vi "Trigger AI Acquisition.vi"() -> ()   [LabVIEW 2012]
doc: "该范例演示了如果使用DAQmx设备连续采集带缓冲的电压信号。\n\n关于如何连接信号至DAQ设备，请查看设备文档。"
uses:
  <vilib>/DAQmx/read.llb/DAQmx Read (Analog 1D Wfm NChan NSamp).vi
  <vilib>/DAQmx/create/channels.llb/DAQmx Create Channel (AI-Voltage-Basic).vi
  <vilib>/DAQmx/configure/timing.llb/DAQmx Timing (Sample Clock).vi
  <vilib>/DAQmx/configure/task.llb/DAQmx Configure Logging (TDMS).vi
  <vilib>/DAQmx/configure/trigger.llb/DAQmx Start Trigger (Digital Edge).vi
  <vilib>/DAQmx/miscellaneous.llb/DAQmx Fill In Error Info.vi
  <resource>/objmgr/daqmx.rc
panel:
  in  "边沿":i32(ring)=10280 items=["上升"=10280, "下降"=10171]
  in  "源":tag="/Dev1/PFI1"
  in  "停止":bool
  out "波形图":waveform(dbl)[](graph)=[{"t0"=timestamp(3423073651.7132955 s since 1904-01-01), "dt"=0.001, "Y"=array[1000 elements], "attributes"=variant("NI_ChannelName"=variant(string "Dev1/ai1"), "NI_UnitDescription"=variant(string "Volts"))}]
  in  "TDMS文件路径":path
  in  "每个循环采样点":i32=1000
  in  "采样率":dbl=1000.0
  in  "采样时钟源":tag="OnboardClock"
  in  "接线端配置":i32(ring)=-1 items=["默认"=-1, "RSE"=10083, "NRSE"=10078, "差分"=10106, "伪差分"=12529]
  in  "最大电压":dbl=1.0
  in  "最小电压":dbl=-1.0
  in  "物理通道":tag="Dev1/ai1"
  out "实际采样率":dbl=1000.0 format="%0.2f"
  in  "记录模式":i32(ring)=10231 items=["关"=10231, "记录并读取"=15842]
  # "通道设置"
  # "触发设置"
  # "采集数据"
  # "定时设置"
  # "记录设置"
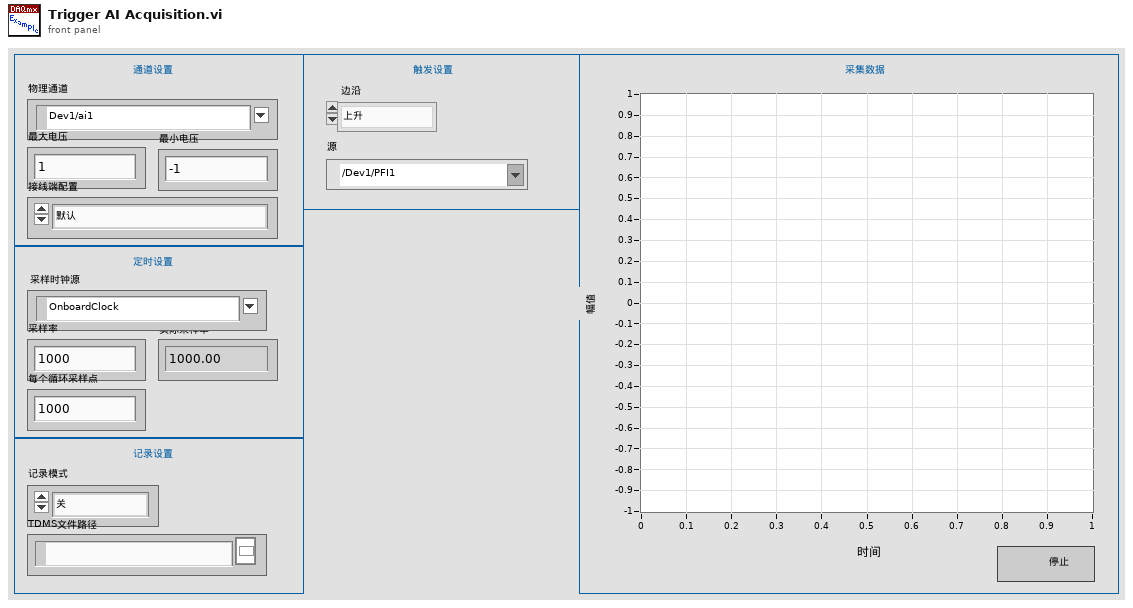
[diagram p1: front panel]
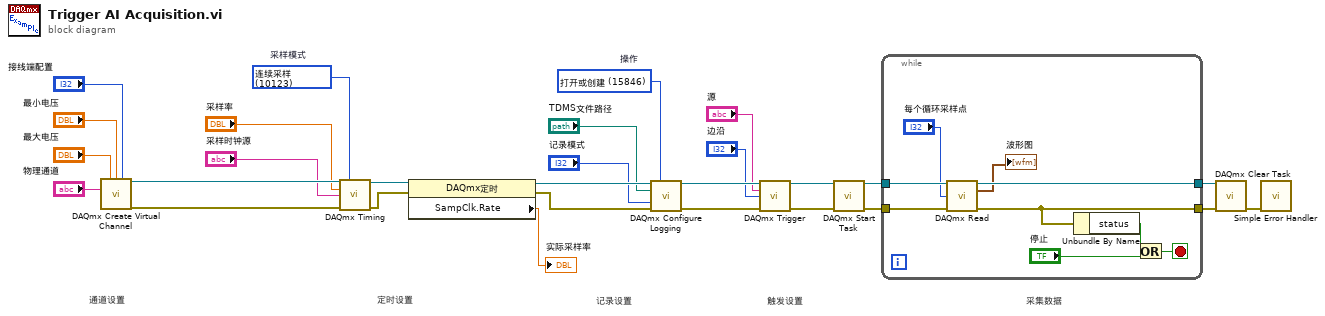
[diagram p0: block diagram]
diagram:
  w1 = 15846 items=["打开"=10437, "打开或创建"=15846, "创建或替换"=15847, "创建"=15848]  # 操作
  w2 = 10123 items=["有限采样"=10178, "连续采样"=10123, "硬件定时单点"=12522]  # 采样模式
  # "触发设置"
  # "采集数据"
  # "定时设置"
  # "通道设置"
  # "记录设置"
  n1 = call-poly <vilib>:"DAQmx Create Virtual Channel.vi"("maximum value"="最大电压", "minimum value"="最小电压", "input terminal configuration"="接线端配置", "physical channels"="物理通道") -> ("task out"=w25:refnum<k21>, "error out"=w26:errorcluster)  [unwired: 10 in]
  n2 = call-poly <vilib>:"DAQmx Timing.vi"("task/channels in"=w25, "sample mode"=w2, "rate"="采样率", "source"="采样时钟源", "error in"=w26) -> ("task out"=w28:refnum<k21>, "error out"=w27:errorcluster)  [unwired: 9 in]
  n3 = property on="属性节点" class="DAQmx定时"(reference=w28, error in=w27) -> (reference out=w24:refnum<k21>, error out=w23:errorcluster, "SampClk.Rate"=→"实际采样率":dbl)
  n4 = call-poly <vilib>:"DAQmx Configure Logging.vi"("task/channels in"=w24, "operation"=w1, "file path"="TDMS文件路径", "logging mode"="记录模式", "error in"=w23) -> ("task out"=w8:refnum<k21>, "error out"=w6:errorcluster)  [unwired: 9 in]
  n5 = call-poly <vilib>:"DAQmx Trigger.vi"("task/channels in"=w8, "source"="源", "edge"="边沿", "error in"=w6) -> ("task out"=w7:refnum<k21>, "error out"=w5:errorcluster)  [unwired: 10 in]
  n6 = call <vilib>:"DAQmx Start Task.vi"("task/channels in"=w7, "error in"=w5) -> ("task out"=w22:refnum<k21>, "error out"=w21:errorcluster)  [unwired: 12 in]
  n7 = while {
    tunnel: w22 -> [w37]
    tunnel: w21 -> [w36]
    tunnel: [w33] -> w19
    tunnel: [w34] -> w20
    stop <- w35 stop-if-true
    n8 = call-poly <vilib>:"DAQmx Read.vi"("task/channels in"=w37, "number of samples per channel"="每个循环采样点", "error in"=w36) -> ("task out"=w34:refnum<k21>, "data"=→"波形图":waveform(dbl)[], "error out"=w33:errorcluster)  [unwired: 10 in]
    n9 = Unbundle By Name ("按名称解除捆绑")(w33) -> ("status"=w32:bool)
    n10 = Or ("或")(x=w32, y="停止") -> (x .or. y?=w35:bool)
  }
  n11 = call <vilib>:"DAQmx Clear Task.vi"("task in"=w20, "error in"=w19) -> ("error out"=w18:errorcluster)  [unwired: 13 in]
  n12 = call <vilib>:"Simple Error Handler.vi"("error in (no error)"=w18) -> ()  [unwired: 4 in, 5 out]
